vi "Save Temperature.vi"(8 "error in (no error)":errorcluster, 11 "Pulse Controller in":refnum<class "Pulse Controller.lvclass">) -> (0 "error out":errorcluster, 3 "Pulse Controller out":refnum<class "Pulse Controller.lvclass">)   [LabVIEW 2024, in "Pulse Controller.lvclass"]
uses:
  Pulse Controller.lvclass
  C:/Git/LabActor/Template Module/Template Module.lvclass
  NHMFL_Core/Libraries/File/Metadata/Metadata.lvclass
  Template Module/Template Module.lvclass/Template Module.ctl
  Template Module/Read Logger.vi
  Template Module/Write Logger.vi
  Loggers/Logger/Logger.lvclass
  Pulse Controller.lvclass/Pulse Controller.ctl
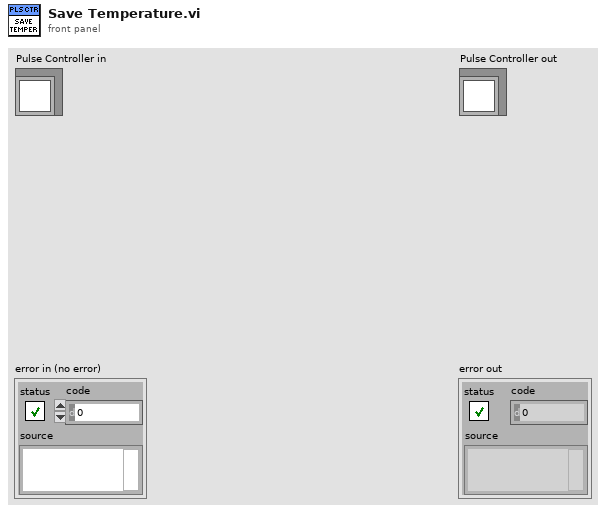
[diagram p1: front panel]
types:
  T1 = cluster{timestamp, "String":string, "String":string}[]
  T2 = cluster{timestamp, "String":string, "String":string}
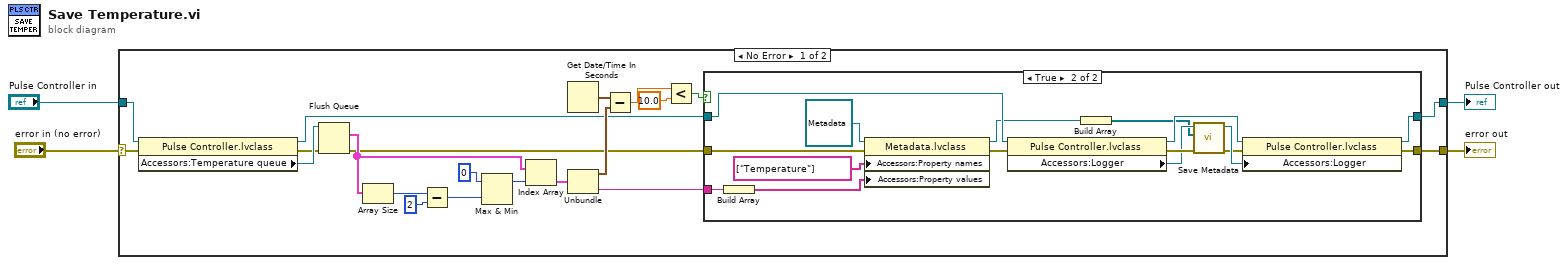
[diagram p0: block diagram]
diagram:
  n1 = case shown="No Error" "error in (no error)" {
    selector: "error in (no error)" -> [w25 w45]
    tunnel: [w8 w45] -> w3
    tunnel: [w5 w44] -> w1
    tunnel: "Pulse Controller in" -> [w24 w44]
    frame No Error {
      n2 = property class="Pulse Controller.lvclass"(reference=w24, error in=w25) -> (reference out=w6:refnum<class "Pulse Controller.lvclass">, error out=w11:errorcluster, "Accessors:Temperature queue"=w23:refnum<queue>)
      n3 = Flush Queue(queue=w23, error in (no error)=w11) -> (remaining elements=w17:T1, error out=w9:errorcluster)  [unwired: 1 out]
      n4 = Array Size(array=w17) -> (size(s)=w22:i32)
      n5 = Subtract(x=w22, y=2) -> (x-y=w20:i32)
      n6 = Max & Min(x=0, y=w20) -> (max(x,y)=w19:i32)  [unwired: 1 out]
      n7 = Index Array(array=w17, index=w19) -> (element=w16:T2)
      n8 = Get Date/Time In Seconds() -> (seconds since 1Jan1904=w15:timestamp)
      n9 = Unbundle(w16) -> (w14:timestamp, "String"=w7:string)  [unwired: 1 out]
      n10 = Subtract(x=w15, y=w14) -> (x-y=w13:dbl)
      n11 = Less?(x=w13, y=10.0) -> (x < y?=w10:bool)
      n12 = case shown="True" w10 {
        tunnel: w9 -> [w26 w33]
        tunnel: [w26 w36] -> w8
        tunnel: w7 -> [_ w29]
        tunnel: w6 -> [w27 w43]
        tunnel: [w27 w37] -> w5
        frame False {
        }
        frame True {
          n13 = Build Array(w29) -> (w28:string[])
          n14 = property class="Metadata.lvclass"(reference=refnum<class "Metadata.lvclass"> refnum ("Metadata.lvclass"), error in=w33, "Accessors:Property names"=string[] ["Temperature"] ("Property names"), "Accessors:Property values"=w28) -> (reference out=w31:refnum<class "Metadata.lvclass">, error out=w32:errorcluster)
          n15 = property class="Pulse Controller.lvclass"(reference=w43, error in=w32) -> (reference out=w38:refnum<class "Pulse Controller.lvclass">, error out=w42:errorcluster, "Accessors:Logger"=w41:refnum<class "Logger.lvclass">)
          n16 = Build Array(w31) -> (w30:refnum<class "Metadata.lvclass">[])
          n17 = call-dynamic "Save Metadata.vi"("error in (no error)"=w42, "Metadata"=w30, "Logger in"=w41) -> ("error out"=w39:errorcluster, "Logger out"=w40:refnum<class "Logger.lvclass">)  [unwired: 5 in, 2 out]
          n18 = property class="Pulse Controller.lvclass"(reference=w38, error in=w39, "Accessors:Logger"=w40) -> (reference out=w37:refnum<class "Pulse Controller.lvclass">, error out=w36:errorcluster)
        }
      }
    }
    frame Error {
    }
  }
  "error out" <- w3
  "Pulse Controller out" <- w1
